vi "Create Stop.vi"(8 "error in (no error)":errorcluster, 11 "Thread in":refnum<class "Thread.lvclass">) -> (0 "error out":errorcluster, 3 "Thread out":refnum<class "Thread.lvclass">)   [LabVIEW 2019, in "DSF Core.lvlib" / "Thread.lvclass"]
uses:
  Thread.lvclass
  <vilib>/NI/Memory Manager/Classes/Pointer/Pointer.lvclass/Pointer.ctl
  Thread.lvclass/Thread.ctl
  <vilib>/NI/Memory Manager/Classes/Pointer/Set Address.vi
  <vilib>/NI/Memory Manager/Classes/Pointer/Set Size.vi
  <vilib>/NI/Memory Manager/Classes/Pointer/Set Internal.vi
  <vilib>/NI/Memory Manager/Classes/Pointer/Pointer.lvclass
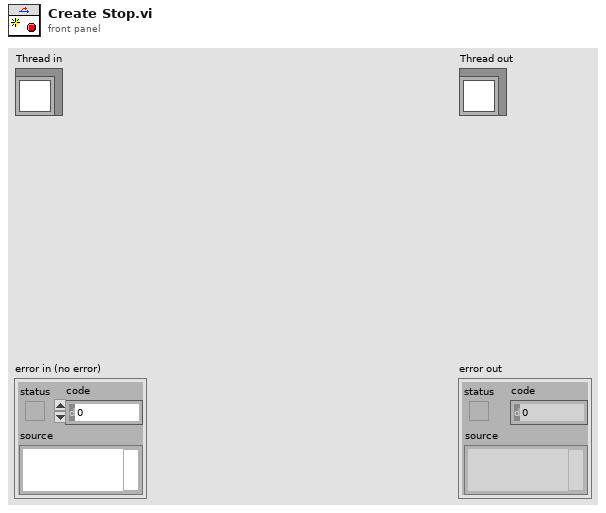
[diagram p1: front panel]
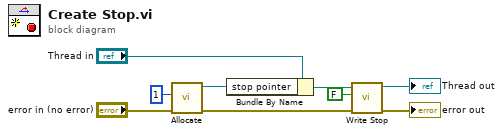
[diagram p0: block diagram]
diagram:
  n1 = call <vilib>:"Allocate.vi"("error in (no error)"="error in (no error)", "size"=u64 1 ("count (1)")) -> ("error out"=w5:errorcluster, "Pointer out"=w7:refnum<class "Pointer.lvclass">)  [unwired: 8 in]
  n2 = Bundle By Name(cluster="Thread in", "stop pointer"=w7) -> (w3:refnum<class "Thread.lvclass">)
  n3 = call "Write Stop.vi"("error in (no error)"=w5, "stop"=FALSE, "Thread in"=w3) -> ("error out"=→"error out":errorcluster, "Thread out"=→"Thread out":refnum<class "Thread.lvclass">)  [unwired: 7 in]
